vi "Calculate_NACA0015_Variables.vi"() -> (0 "New Values In":string[][](array[string])=[["Test data5"]], 1 "New Chs In":string[](array[string])=["30-10-03:New:Channel new5"])   [LabVIEW 2011]
uses:
  Results_plotter_Global.vi
  <vilib>/Analysis/coordinate.llb/2D Cartesian Coordinate Rotation (Scalar).vi
  <vilib>/Analysis/NI_AALPro.lvlib
  <vilib>/Analysis/NI_AALBase.lvlib
panel:
  out "Cp v yc 3":cluster{dbl[], dbl[]}(graph)
  out "Cp v yc 2":cluster{dbl[], dbl[]}(graph)
  out "size(s)":i32
  out "Cp v yc":cluster{dbl[], dbl[]}(graph)
  out "Cl":dbl
  out "Cd":dbl
  out "Legend of ch names":string[](array[string])
  out "Cp v xc":cluster{dbl[], dbl[]}(graph)
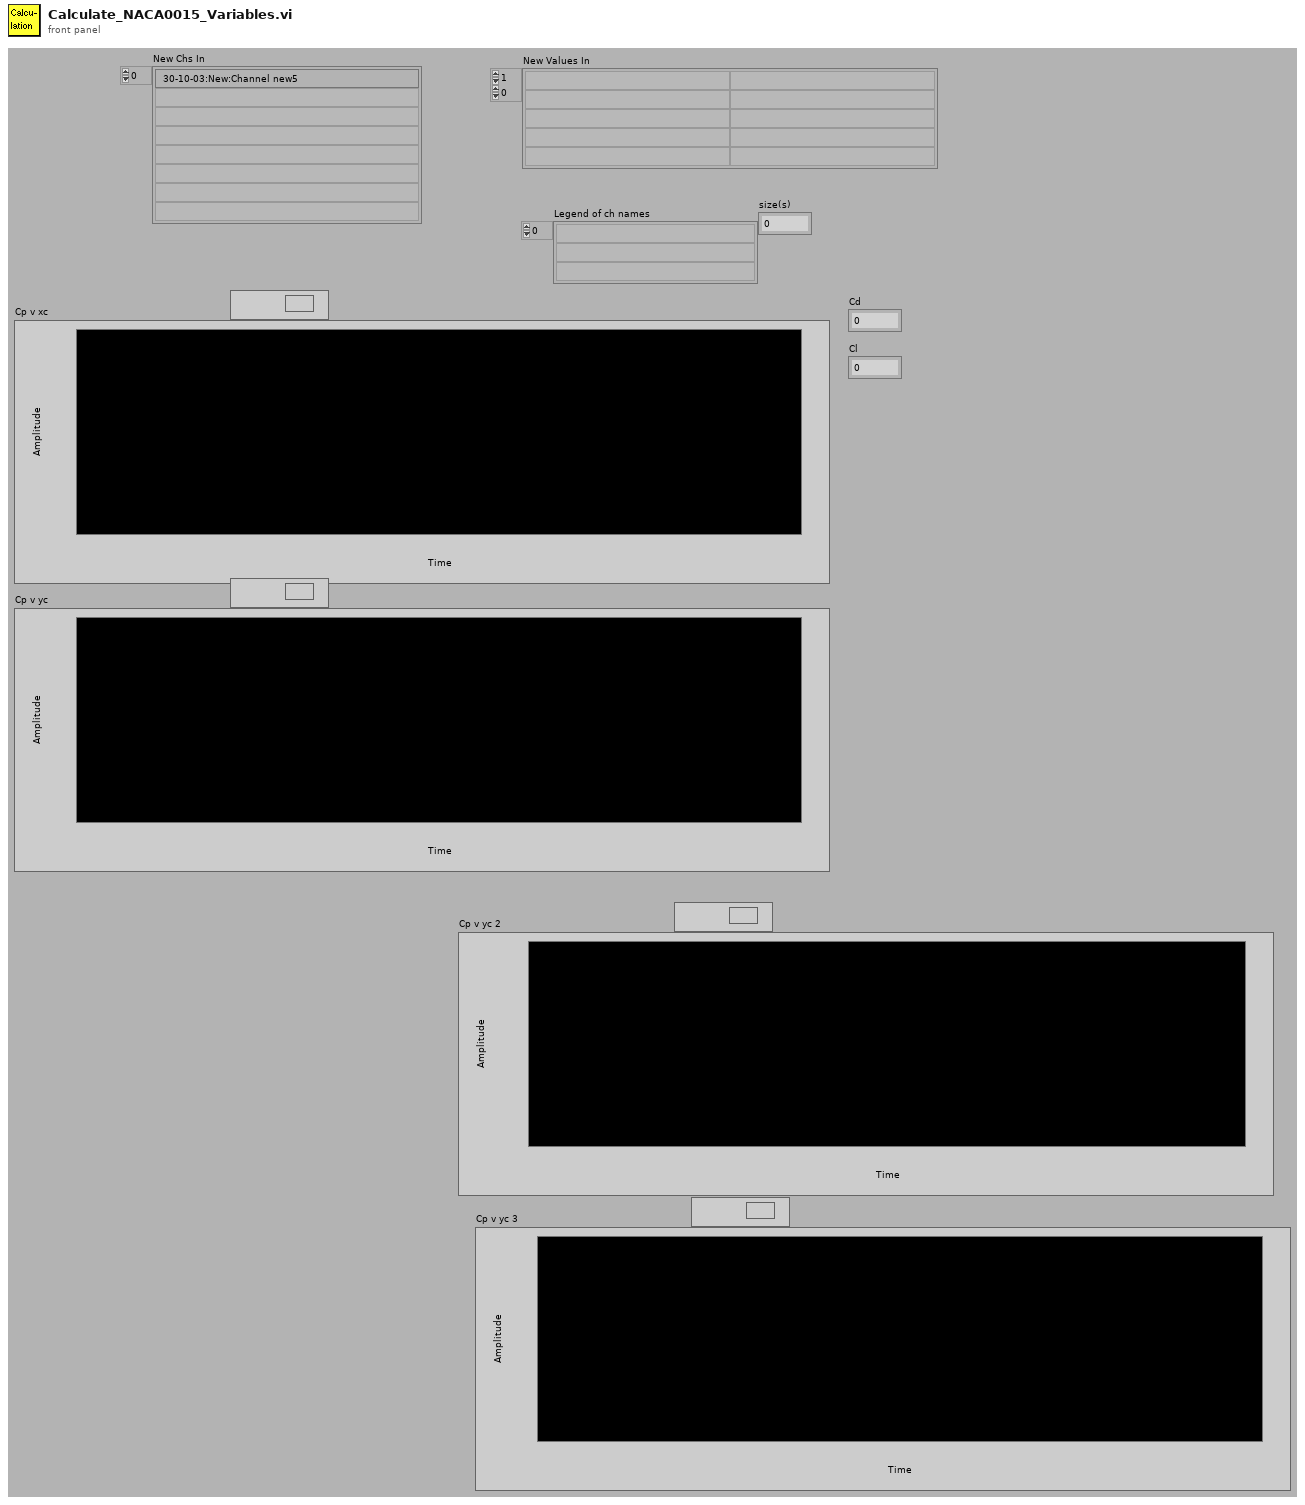
[diagram p1: front panel]
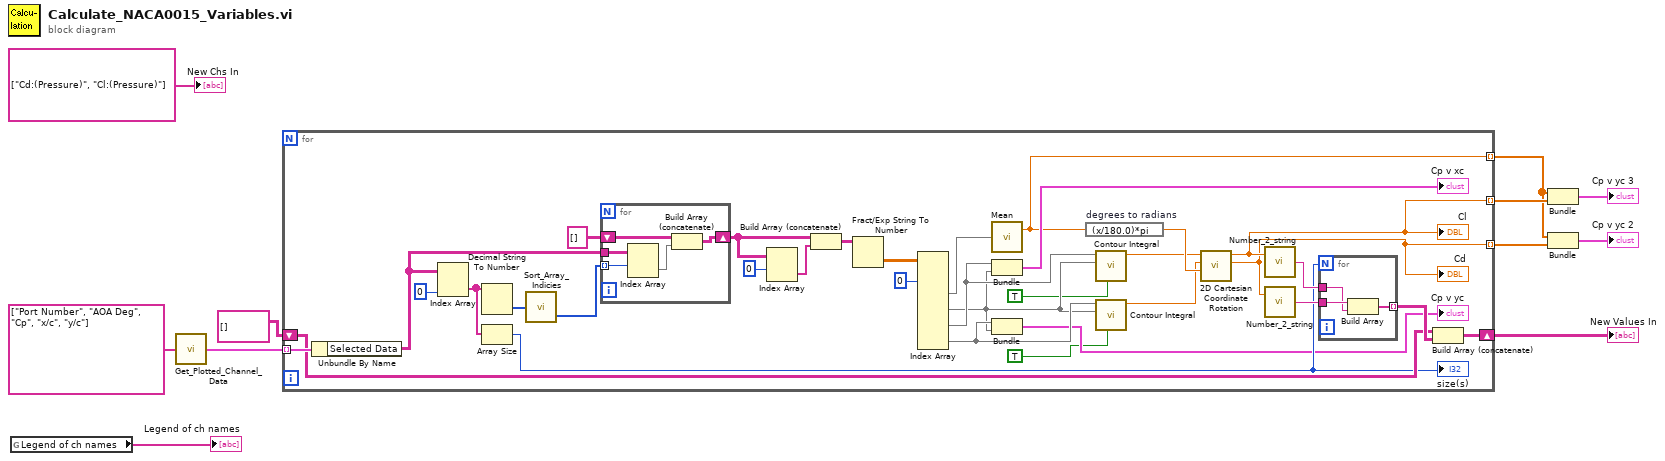
[diagram p0: block diagram]
diagram:
  n1 = global read "Results_plotter_Global.vi" "Legend of ch names"() -> (→"Legend of ch names":string[])
  n2 = call "Get_Plotted_Channel_Data.vi"("Channel Names"=string[] ["Port Number", "AOA Deg", "Cp", "x/c", "y/c"]) -> ("Selected Data Cluster"=w11:cluster{"Selected Data":string[][]}[])  [unwired: 4 in]
  n3 = for {
    tunnel: w11 -> [w43] mode=indexing
    shift-right: [w39] -> w1
    shift-left: string[][] [] -> [w38]
    tunnel: [w14] -> w7 mode=indexing
    tunnel: [w13] -> w5 mode=indexing
    tunnel: [w12] -> w6 mode=indexing
    n4 = Unbundle By Name(w43) -> ("Selected Data"=w26:string[][])
    n5 = Index Array(array=w26, index (col)=0 ("disabled index (col)")) -> (element=w35:string[])  [unwired: 1 in]
    n6 = Decimal String To Number(string=w35) -> (number=w36:i32[])  [unwired: 2 in, 1 out]
    n7 = Array Size(array=w35) -> (size(s)=w34:i32)
    "size(s)" <- w34
    n8 = call "Sort_Array_Indicies.vi"("unsorted array"=w36) -> ("Sort Index"=w33:i32[])  [unwired: 1 out]
    n9 = for {
      tunnel: w26 -> [w49]
      tunnel: w33 -> [w48] mode=indexing
      shift-right: [w45] -> w31
      shift-left: string[][] [] -> [w46]
      n10 = Index Array(array=w49, index (row)=w48) -> (element=w47:string[])  [unwired: 1 in]
      n11 = Build Array (concatenate)(w46, w47) -> (w45:string[][])
    }
    n12 = Index Array(array=w31, index (row)=0 ("disabled index (col)")) -> (element=w30:string[])  [unwired: 1 in]
    n13 = Build Array (concatenate)(w31, w30) -> (w29:string[][])
    n14 = Fract/Exp String To Number(string=w29) -> (number=w21:dbl[][])  [unwired: 3 in, 1 out]
    n15 = Index Array(array=w21, index (col) #1=0 ("disabled index (col)")) -> (element #2=w28:dbl[], element #3=w17:dbl[], element #4=w18:dbl[], element #5=w27:dbl[])  [unwired: 9 in, 1 out]
    n16 = call <vilib>:"Mean.vi"("X"=w28) -> ("mean"=w12:dbl)  [unwired: 1 out]
    n17 = Bundle(w18, w17) -> (→"Cp v xc":cluster{dbl[], dbl[]})  [unwired: 1 in]
    n18 = Bundle(w27, w17) -> (→"Cp v yc":cluster{dbl[], dbl[]})  [unwired: 1 in]
    n19 = expression code="(x/180.0)*pi" "degrees to radians"(w12) -> (w44:dbl)
    n20 = call "Contour Integral.vi"("Reverse direction?"=TRUE, "Y"=w17, "X"=w18) -> ("Integral of Y"=w20:dbl)  [unwired: 8 in]
    n21 = call "Contour Integral.vi"("Reverse direction?"=TRUE, "Y"=w17, "X"=w27) -> ("Integral of Y"=w19:dbl)  [unwired: 8 in]
    n22 = call-poly <vilib>:"2D Cartesian Coordinate Rotation.vi"("theta"=w44, "y"=w19, "x"=w20) -> ("y out"=w13:dbl, "x out"=w14:dbl)  [unwired: 6 in, 1 out]
    "Cd" <- w13
    "Cl" <- w14
    n23 = call "Number_2_string.vi"("number"=w14) -> ("String"=w42:string)  [unwired: 1 in]
    n24 = call "Number_2_string.vi"("number"=w13) -> ("String"=w41:string)  [unwired: 1 in]
    n25 = for {
      N: w34 -> [_]
      tunnel: w41 -> [w52]
      tunnel: [w51] -> w40 mode=indexing
      tunnel: w42 -> [w50]
      n26 = Build Array(w52, w50) -> (w51:string[])
    }
    n27 = Build Array (concatenate)(w38, w40) -> (w39:string[][])
  }
  "New Values In" <- w1
  n28 = Bundle(w6, w7) -> (→"Cp v yc 3":cluster{dbl[], dbl[]})  [unwired: 1 in]
  n29 = Bundle(w6, w5) -> (→"Cp v yc 2":cluster{dbl[], dbl[]})  [unwired: 1 in]
  "New Chs In" <- string[] ["Cd:(Pressure)", "Cl:(Pressure)"] ("Channel Names")
